vi "DTHPHW_OpcuaServer.vi"() -> ()   [LabVIEW 2024]
panel:
  out "Error Closing Server":errorcluster
  in  "Error Opening Server":errorcluster
  # "****** SERVER  OPC UA DEMARRE  *********\n\nDemarrage du serveur : AUTOMATIQUE\nArrêt du serveur : SORTIR DE L'APPLICATION"
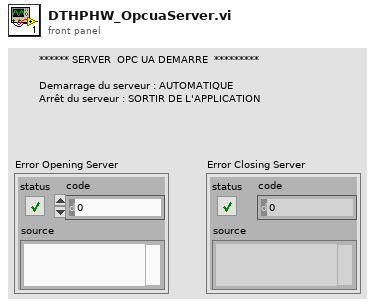
[diagram p1: front panel]
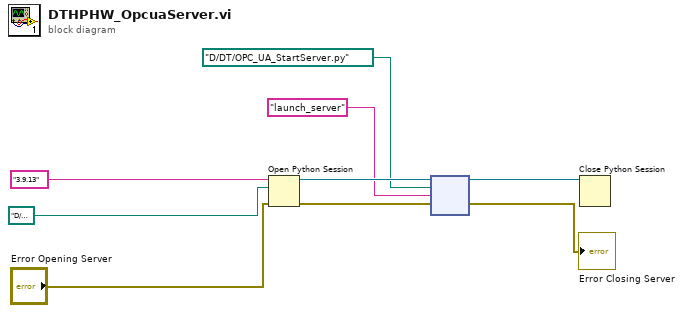
[diagram p0: block diagram]
diagram:
  n1 = Open Python Session(python version="3.9.13" ("Python version"), python path=path "D:/Python/Python39-32/python.exe" ("Python path"), 3:"Error Opening Server") -> (session out=w9:refnum<k35>, error out=w2:errorcluster)
  n2 = node(w9, path "D:/DT/OPC_UA_StartServer.py" ("module path"), "launch_server" ("function name"), w2) -> (w7:refnum<k35>, →"Error Closing Server":errorcluster)  [unwired: 2 in, 2 out]
  n3 = Close Python Session(session in=w7) -> ()  [unwired: 1 in, 1 out]
